vi "Add clue to error cluster.vi"(8 "error in (no error)":errorcluster, 11 "String":string) -> (0 "error out":errorcluster)   [LabVIEW 2020, in "TOML.lvlib"]
uses:
  TOML.lvlib
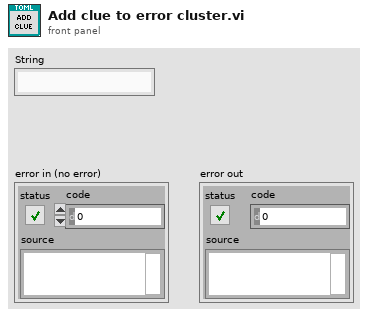
[diagram p1: front panel]
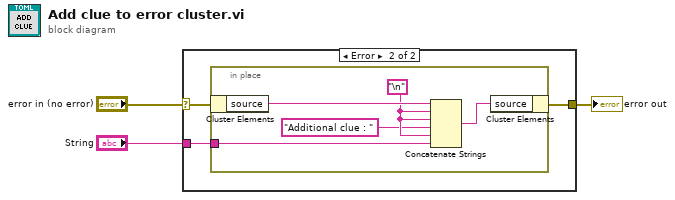
[diagram p0: block diagram]
diagram:
  n1 = case shown="Error" "error in (no error)" {
    selector: "error in (no error)" -> [w4 w7]
    tunnel: [w4 w6] -> w3
    tunnel: "String" -> [_ w5]
    frame No Error {
    }
    frame Error {
      n2 = in-place {
        in-place-border: w5 -> [w8]
        w10 = "\n"
        n3 = in-place-cluster #1(w7) -> ("source"=w12:string)
        n4 = Concatenate Strings(w12, w10, w10, "Additional clue : " ("string"), w10, w8) -> (w11:string)
        n5 = in-place-cluster #1("source"=w11) -> (w6:errorcluster)
      }
    }
  }
  "error out" <- w3
